vi "TCP-Generic Ack.vi"(0 "connection ID":refnum<k5>, 3 "error in (no error)":errorcluster) -> (7 "connection ID out":refnum<k5>, 10 "error out":errorcluster)   [LabVIEW 2020]
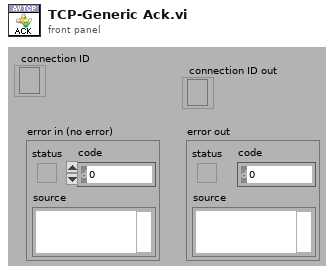
[diagram p1: front panel]
types:
  T1 = enum16{"big-endian, network order", "native, host order", "little-endian"}
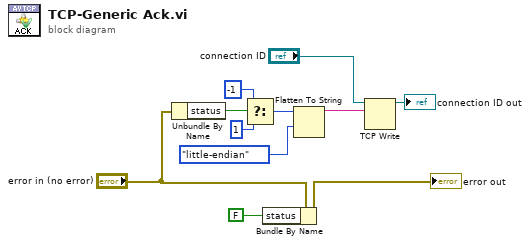
[diagram p0: block diagram]
diagram:
  n1 = Unbundle By Name("error in (no error)") -> ("status"=w10:bool)
  n2 = Select(t=-1, s=w10, f=1) -> (s? t:f=w3:i32)
  n3 = Bundle By Name(cluster="error in (no error)", "status"=FALSE) -> (→"error out":errorcluster)
  n4 = Flatten To String(anything=w3, byte order (0:big-endian, network order)=T1."little-endian") -> (data string=w1:string)  [unwired: 2 in, 2 out]
  n5 = TCP Write(connection ID="connection ID", data in=w1) -> (connection ID out=→"connection ID out":refnum<k5>)  [unwired: 2 in, 2 out]
